vi "Lab.05_DAQ_4.vi"() -> ()   [LabVIEW 2016]
uses:
  <vilib>/Analysis/NI_AAL_SigProc.lvlib
  <vilib>/Analysis/NI_AALPro.lvlib
panel:
  out "derivative in a period":dbl[](graph)
  out "baseline=0.63 of Vpp":dbl[](graph)
  out "time const.":dbl
  out "one period signal":dbl[](graph)
  out "period":dbl
  out "valleys":dbl
  out "peaks":dbl
  out "Min":dbl
  out "Max":dbl
  out "peak to peak amplitude":dbl
  out "input signals":dynamicdata(graph)
  in  "stop":bool
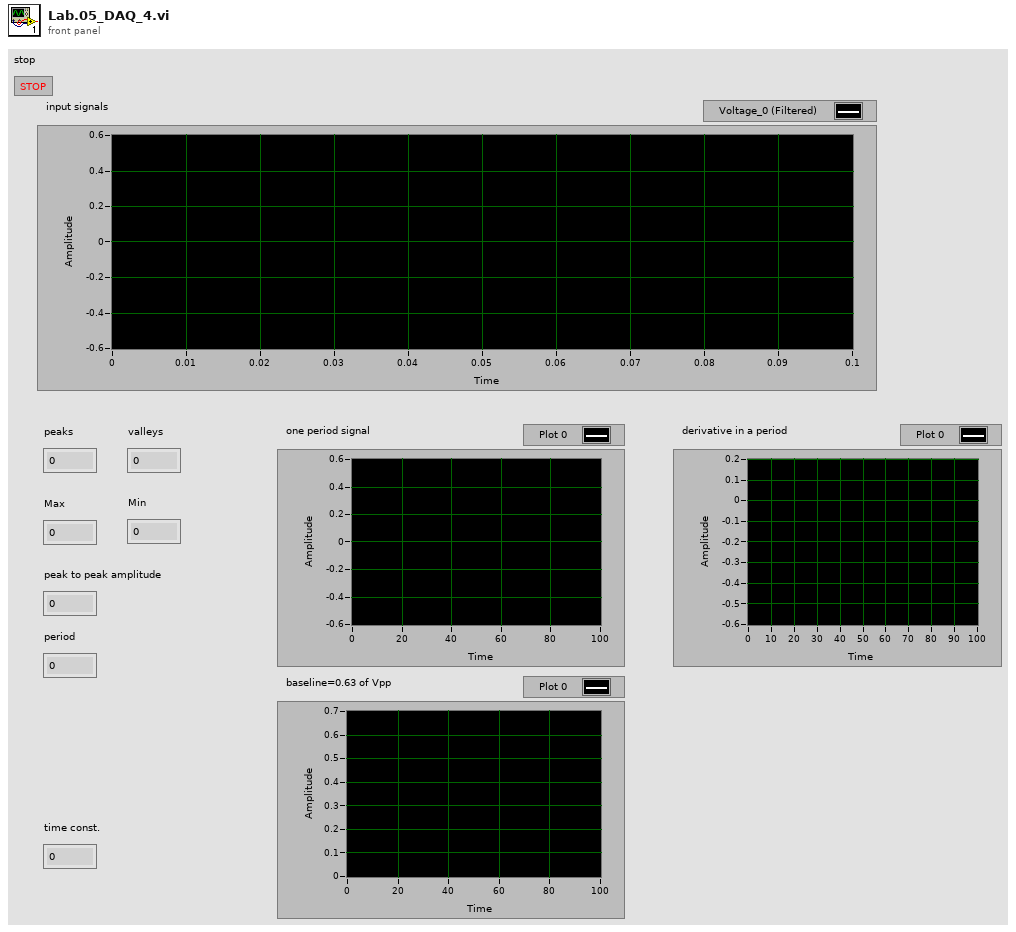
[diagram p1: front panel]
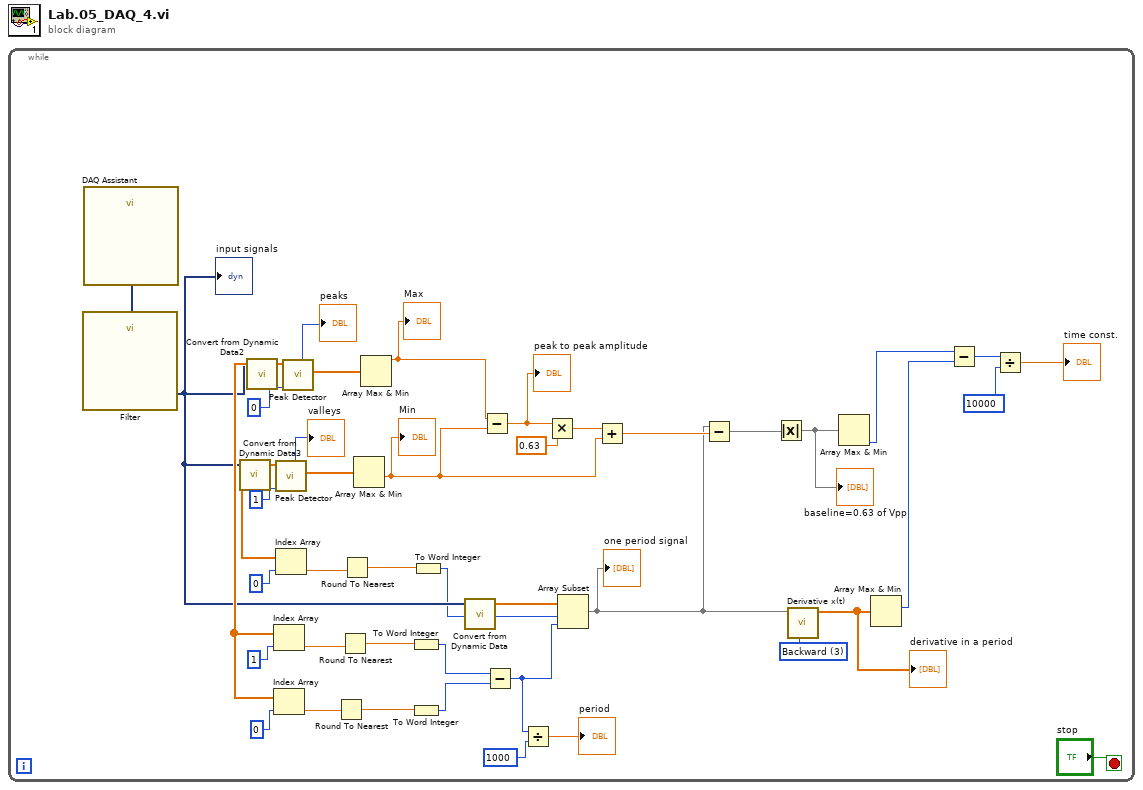
[diagram p0: block diagram]
diagram:
  n1 = while {
    stop <- "stop" stop-if-true
    w13 = u16 3 items=["2nd Order Central", "4th Order Central", "Forward", "Backward"] ("method")
    n2 = call "DAQ Assistant"() -> ("data"=w5:dynamicdata)  [unwired: 16 in, 3 out]
    n3 = call "Filter"("Signal"=w5) -> ("Filtered Signal"=w4:dynamicdata)  [unwired: 9 in, 1 out]
    "input signals" <- w4
    n4 = call "Convert from Dynamic Data3"("Dynamic Data Type"=w4) -> ("Array"=w42:dbl[])  [unwired: 3 in]
    n5 = call "Convert from Dynamic Data2"("Dynamic Data Type"=w4) -> ("Array"=w44:dbl[])  [unwired: 3 in]
    n6 = call <vilib>:"Peak Detector.vi"("peaks/valleys"=1, "X"=w42) -> ("Amplitudes"=w39:dbl[], "Locations"=w20:dbl[], "# found"=→"valleys":i32)  [unwired: 5 in, 2 out]
    n7 = Index Array(array=w20, index=0) -> (element=w22:dbl)
    n8 = call <vilib>:"Peak Detector.vi"("peaks/valleys"=0, "X"=w44) -> ("Amplitudes"=w40:dbl[], "Locations"=w34:dbl[], "# found"=→"peaks":i32)  [unwired: 5 in, 2 out]
    n9 = Index Array(array=w34, index=1) -> (element=w30:dbl)
    n10 = Index Array(array=w34, index=0) -> (element=w32:dbl)
    n11 = Round To Nearest(number=w32) -> (nearest integer value=w31:dbl)
    n12 = Round To Nearest(number=w30) -> (nearest integer value=w29:dbl)
    n13 = Round To Nearest(number=w22) -> (nearest integer value=w21:dbl)
    n14 = Array Max & Min(array=w39) -> (min value=w17:dbl)  [unwired: 3 out]
    "Min" <- w17
    n15 = Array Max & Min(array=w40) -> (max value=w38:dbl)  [unwired: 3 out]
    "Max" <- w38
    n16 = To Word Integer(number=w29) -> (16bit integer=w28:i16)
    n17 = To Word Integer(number=w31) -> (16bit integer=w26:i16)
    n18 = To Word Integer(number=w21) -> (16bit integer=w3:i16)
    n19 = call "Convert from Dynamic Data"("Dynamic Data Type"=w4) -> ("Array"=w27:dbl[])  [unwired: 3 in]
    n20 = Subtract(x=w38, y=w17) -> (x-y=w19:dbl)
    "peak to peak amplitude" <- w19
    n21 = Subtract(x=w28, y=w26) -> (x-y=w2:i16)
    n22 = Divide(x=w2, y=1000) -> (x/y=→"period":dbl)
    n23 = Multiply(x=w19, y=0.63) -> (x*y=w16:dbl)
    n24 = Array Subset(array=w27, index=w3, length=w2) -> (w1:dbl[])
    "one period signal" <- w1
    n25 = Add(x=w16, y=w17) -> (x+y=w15:dbl)
    n26 = Subtract(x=w1, y=w15) -> (x-y=w14:dbl[])
    n27 = Absolute Value(x=w14) -> (abs(x)=w9:dbl[])
    "baseline=0.63 of Vpp" <- w9
    n28 = call <vilib>:"Derivative x(t).vi"("method"=w13, "X"=w1) -> ("dX/dt"=w8:dbl[])  [unwired: 8 in, 1 out]
    "derivative in a period" <- w8
    n29 = Array Max & Min(array=w9) -> (min index (indices)=w7:i32)  [unwired: 3 out]
    n30 = Array Max & Min(array=w8) -> (max index (indices)=w6:i32)  [unwired: 3 out]
    n31 = Subtract(x=w7, y=w6) -> (x-y=w12:i32)
    n32 = Divide(x=w12, y=10000) -> (x/y=→"time const.":dbl)
  }
